vi "Kelompok 3_Case Structure.vi"() -> ()   [LabVIEW 2020]
panel:
  in  "Numeric":i32
  in  "Fahrenheit 2":dbl(slide) scale=0.0..200.0
  out "Celsius 2":dbl(slide) scale=0.0..100.0
  out "Kelvin 2":dbl(slide) scale=250.0..350.0
  in  "stop 2":bool
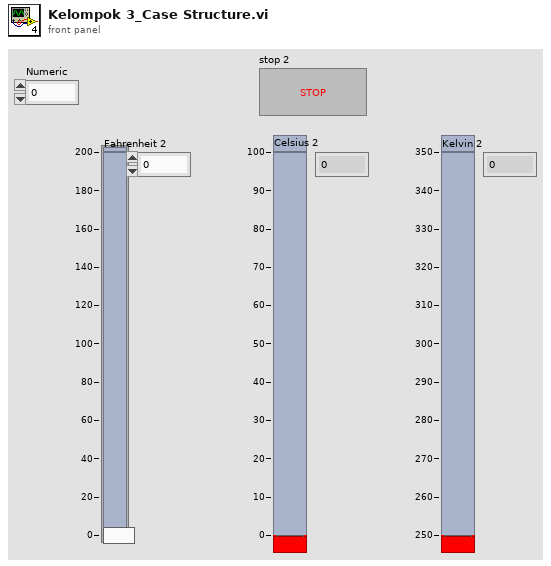
[diagram p1: front panel]
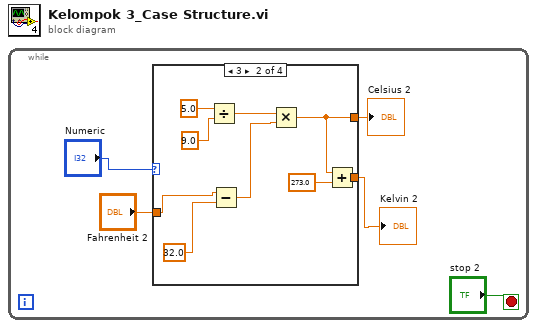
[diagram p0: block diagram]
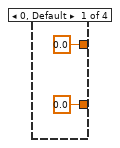
[diagram p2: hidden frame]
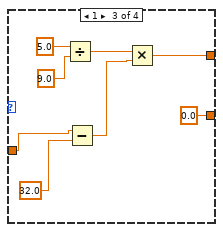
[diagram p3: hidden frame]
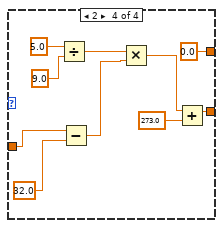
[diagram p4: hidden frame]
diagram:
  n1 = while {
    stop <- "stop 2" stop-if-true
    n2 = case shown="3" "Numeric" {
      tunnel: [0.0 w16 w18 0.0] -> w5
      tunnel: [0.0 w15 0.0 w26] -> w4
      tunnel: "Fahrenheit 2" -> [_ w14 w24 w27]
      frame 0, Default {
      }
      frame 3 {
        n3 = Divide(x=5.0, y=9.0) -> (x/y=w12:dbl)
        n4 = Subtract(x=w14, y=32.0) -> (x-y=w13:dbl)
        n5 = Multiply(x=w12, y=w13) -> (x*y=w16:dbl)
        n6 = Add(x=w16, y=273.0) -> (x+y=w15:dbl)
      }
      frame 1 {
        n7 = Divide(x=5.0, y=9.0) -> (x/y=w22:dbl)
        n8 = Subtract(x=w24, y=32.0) -> (x-y=w23:dbl)
        n9 = Multiply(x=w22, y=w23) -> (x*y=w18:dbl)
      }
      frame 2 {
        n10 = Divide(x=5.0, y=9.0) -> (x/y=w32:dbl)
        n11 = Subtract(x=w27, y=32.0) -> (x-y=w33:dbl)
        n12 = Multiply(x=w32, y=w33) -> (x*y=w34:dbl)
        n13 = Add(x=w34, y=273.0) -> (x+y=w26:dbl)
      }
    }
    "Celsius 2" <- w5
    "Kelvin 2" <- w4
  }
